vi "OurFirstVI.vi"() -> ()   [LabVIEW 2015]
panel:
  out "Num3":dbl
  in  "Num2":dbl
  in  "Num1":dbl
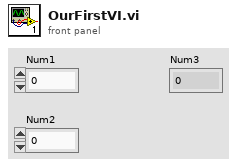
[diagram p1: front panel]
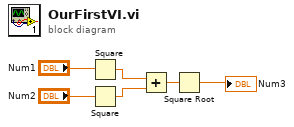
[diagram p0: block diagram]
diagram:
  n1 = Square(x="Num1") -> (x^2=w3:dbl)
  n2 = Square(x="Num2") -> (x^2=w2:dbl)
  n3 = Add(x=w3, y=w2) -> (x+y=w4:dbl)
  n4 = Square Root(x=w4) -> (sqrt(x)=→"Num3":dbl)
